vi "Read Holding Registers.vi"(8 "error in":errorcluster, 9 "number of registers":u16, 10 "starting address":u16, 11 "Standard Data Model in":refnum<class "Standard Data Model.lvclass">) -> (0 "error out":errorcluster, 2 "data":u16[](array[numeric]), 3 "Standard Data Model out":refnum<class "Standard Data Model.lvclass">)   [LabVIEW 2013, in "Modbus Library - Advance.lvlib" / "Standard Data Model.lvclass"]
doc: "Reads N holding registers from the device model, starting at register M."
uses:
  Standard Data Model.lvclass
  Standard Data Model.lvclass/Standard Data Model.ctl
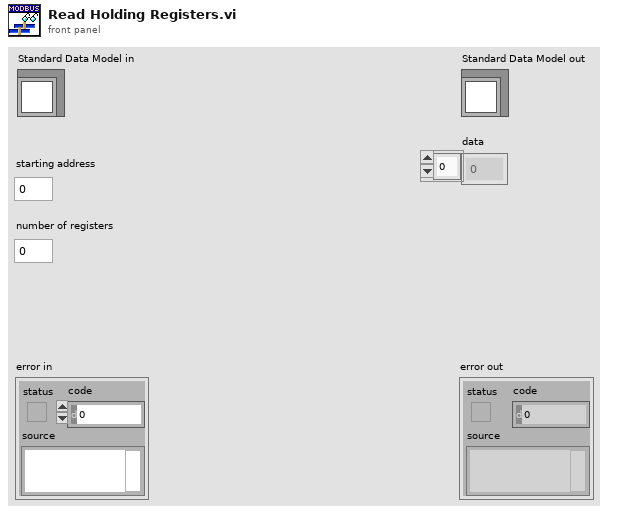
[diagram p1: front panel]
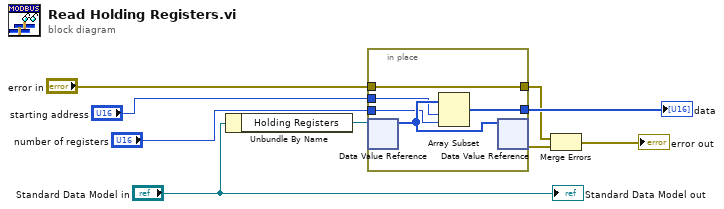
[diagram p0: block diagram]
diagram:
  n1 = Unbundle By Name("Standard Data Model in") -> ("Holding Registers"=w6:refnum<data-value>)
  n2 = in-place {
    in-place-border: "error in" -> [w14]
    in-place-border: [w14] -> w1
    in-place-border: [w13] -> w5
    in-place-border: "starting address" -> [w11]
    in-place-border: "number of registers" -> [w10]
    n3 = in-place-dvr #1(w6) -> (w12:u16[])  [unwired: 1 out]
    n4 = Array Subset(array=w12, index=w11, length=w10) -> (w13:u16[])
    n5 = in-place-dvr #1(w12) -> (w2:errorcluster)  [unwired: 1 out]
  }
  "data" <- w5
  n6 = Merge Errors(w1, w2) -> (→"error out":errorcluster)
  "Standard Data Model out" <- "Standard Data Model in"
